vi "I2C Set Output Enabled.vi"(8 "error in (no error)":errorcluster, 10 "Output Enabled (T:Enable)":bool=TRUE, 11 "Task In":refnum<k21>) -> (0 "error out":errorcluster, 3 "Task Out":refnum<k21>)   [LabVIEW 2017, in "I2C.lvlib"]
doc: "Enables or disables the specific digital output."
uses:
  <vilib>/robotics/Protocols/I2C/DAQmx/I2C.lvlib
  <vilib>/DAQmx/write.llb/DAQmx Write (Digital Bool 1Line 1Point).vi
  <vilib>/DAQmx/miscellaneous.llb/DAQmx Fill In Error Info.vi
  <resource>/objmgr/daqmx.rc
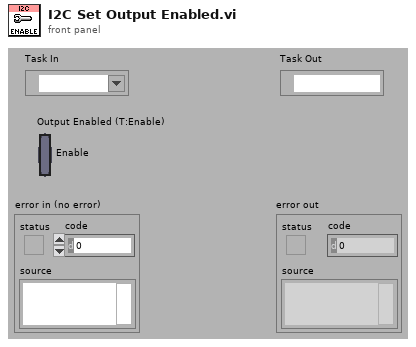
[diagram p1: front panel]
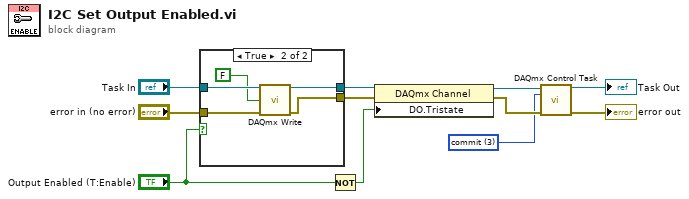
[diagram p0: block diagram]
diagram:
  w6 = 3 items=["verify"=2, "reserve"=4, "commit"=3, "unreserve"=5, "abort"=6] ("action")
  n1 = case shown="True" "Output Enabled (T:Enable)" {
    tunnel: "Task In" -> [w13 w18]
    tunnel: "error in (no error)" -> [w12 w17]
    tunnel: [w13 w15] -> w2
    tunnel: [w12 w14] -> w1
    frame False {
    }
    frame True {
      n2 = call-poly <vilib>:"DAQmx Write.vi"("task/channels in"=w18, "data"=FALSE, "error in"=w17) -> ("task out"=w15:refnum<k21>, "error out"=w14:errorcluster)  [unwired: 10 in, 1 out]
    }
  }
  n3 = Not(x="Output Enabled (T:Enable)") -> (.not. x?=w11:bool)
  n4 = property class="DAQmx Channel"(reference=w2, error in=w1, "DO.Tristate"=w11) -> (reference out=w10:refnum<k21>, error out=w9:errorcluster)
  n5 = call <vilib>:"DAQmx Control Task.vi"("task/channels in"=w10, "action"=w6, "error in"=w9) -> ("task out"=→"Task Out":refnum<k21>, "error out"=→"error out":errorcluster)  [unwired: 11 in]
